vi "Print.vi"(8 "error in":errorcluster, 11 "OD Entry in":refnum<class "OD Entry.lvclass">) -> (0 "error out":errorcluster, 2 "Entry with Sub-Entries":map{string, string}[](array[numeric]), 3 "OD Entry out":refnum<class "OD Entry.lvclass">)   [LabVIEW 2024, in "EDS.lvlib" / "OD Entry.lvclass"]
uses:
  OD Entry.lvclass
  OD Sub-Entry/OD Sub-Entry.lvclass
  D:/git/EDS-File-Viewer/Core/OD Entry/OD Entry.lvclass
  Object Type/Object Type Base.lvclass
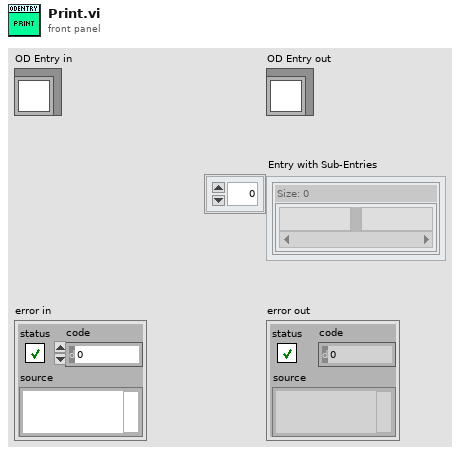
[diagram p1: front panel]
types:
  T1 = typedef "EDS.lvlib/OD Entry.lvclass/ObjectAttributes.ctl" = cluster{"Index":u16, "ObjectType":refnum<class "Object Type Base.lvclass">, "Denotation":string, "Count":u8, "ObjExtend":u8, "PDOtype":T2, "Label":string, "Description":string, "Sub-Entries":map{u16, refnum<class "OD Sub-Entry.lvclass">}}
  T2 = typedef "EDS.lvlib/PDO Mapping Type.ctl" = enum16{"NO", "OPTIONAL", "RPDO", "TPDO", "DEFAULT"}
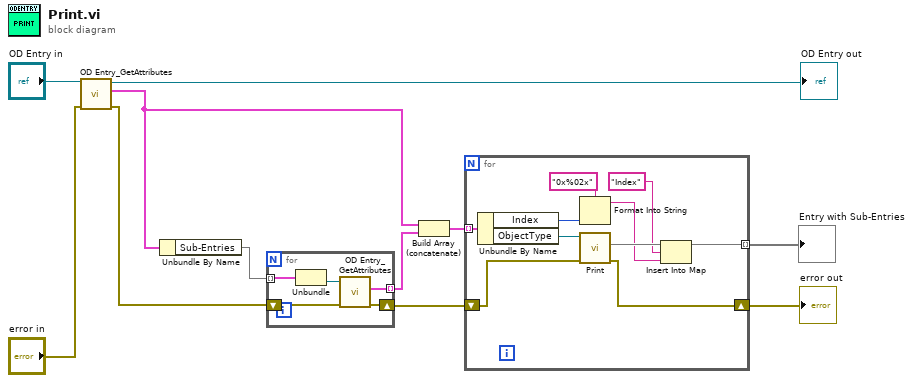
[diagram p0: block diagram]
diagram:
  n1 = call "OD Entry_GetAttributes.vi"("Error In"="error in", "reference in"="OD Entry in") -> ("Error Out"=w7:errorcluster, "Data"=w6:T1, "reference out"=→"OD Entry out":refnum<class "OD Entry.lvclass">)  [unwired: 6 in, 1 out]
  n2 = Unbundle By Name(w6) -> ("Sub-Entries"=w8:map{u16, refnum<class "OD Sub-Entry.lvclass">})
  n3 = for {
    tunnel: w8 -> [w16] mode=indexing
    tunnel: [w13] -> w5 mode=indexing
    shift-right: [w12] -> w3
    shift-left: w7 -> [w14]
    n4 = Unbundle(w16) -> ("OD Sub-Entry"=w15:refnum<class "OD Sub-Entry.lvclass">)  [unwired: 1 out]
    n5 = call "OD Entry_GetAttributes.vi"("Error In"=w14, "reference in"=w15) -> ("Error Out"=w12:errorcluster, "Data"=w13:T1)  [unwired: 6 in, 2 out]
  }
  n6 = Build Array (concatenate)(w6, w5) -> (w4:T1[])
  n7 = for {
    tunnel: w4 -> [w25] mode=indexing
    shift-right: [w17] -> w1
    shift-left: w3 -> [w18]
    tunnel: [w19] -> w2 mode=indexing
    n8 = Unbundle By Name(w25) -> ("Index"=w24:u16, "ObjectType"=w23:refnum<class "Object Type Base.lvclass">)
    n9 = Format Into String(format string="0x%02x", w24) -> (resulting string=w21:string)  [unwired: 2 in, 1 out]
    n10 = call-dynamic "Print.vi"("error in"=w18, "Object Type Base in"=w23) -> ("error out"=w17:errorcluster, "Fields"=w22:map{string, string})  [unwired: 7 in, 1 out]
    n11 = Insert Into Map(map in=w22, key="Index", value=w21) -> (map out=w19:map{string, string})  [unwired: 2 out]
  }
  "error out" <- w1
  "Entry with Sub-Entries" <- w2
